vi "YokoGS200 CheckStatus.vi"(8 "error in (no error)":errorcluster, 11 "VISA Rsrc":refnum<visa-resource-name>="SR530") -> (0 "error out":errorcluster, 1 "Octet d'état":bool[](array[boolean]), 2 "octet d'état":u16, 3 "VISA Rsrc Out":refnum<visa-resource-name>="GPIB0::12::INSTR")   [LabVIEW 2012]
uses:
  <userlib>/Yoko GS200/YokoGS200 lvl_states ctl.ctl
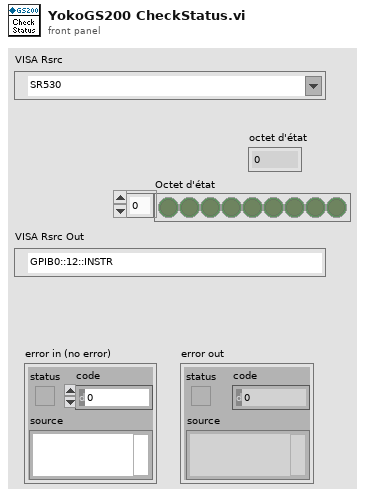
[diagram p1: front panel]
types:
  T1 = typedef "YokoGS200 lvl_states ctl.ctl" = enum16{"RampStep", "Send Command", "Check Errors", "End"}
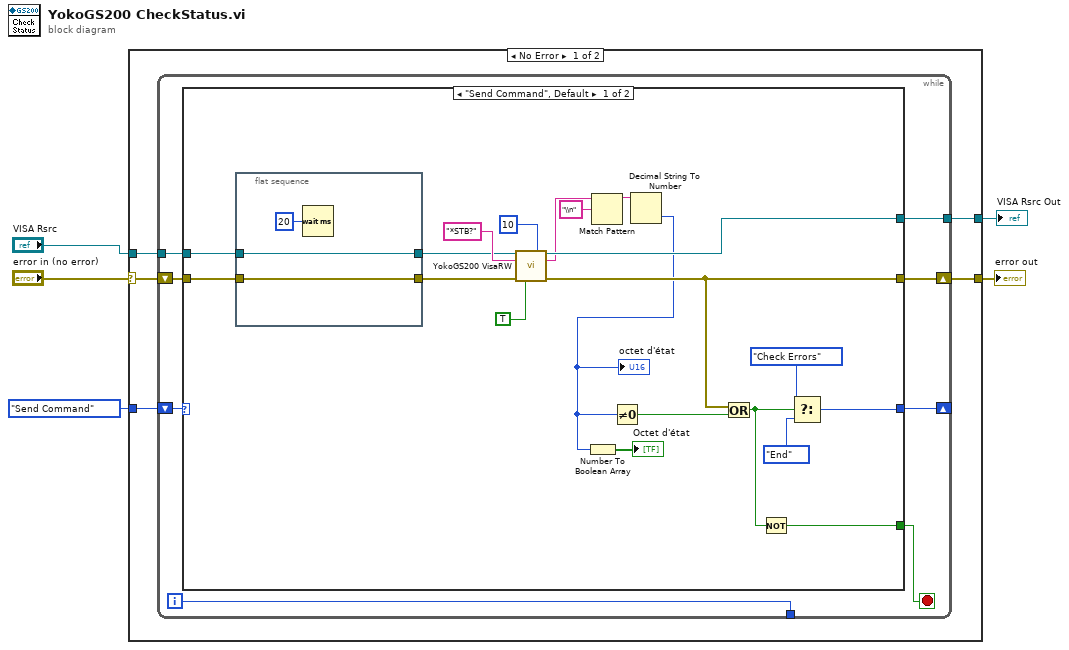
[diagram p0: block diagram]
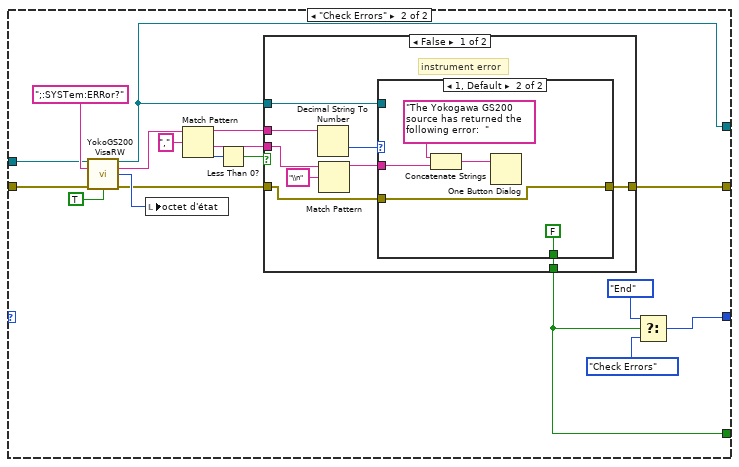
[diagram p2: hidden frame]
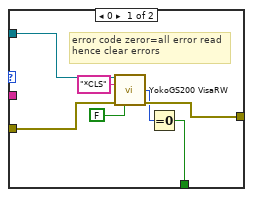
[diagram p3: hidden frame]
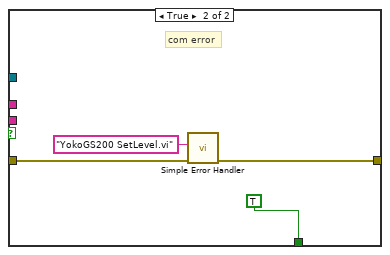
[diagram p4: hidden frame]
diagram:
  n1 = case shown="No Error" "error in (no error)" {
    selector: "error in (no error)" -> [w10 w85]
    tunnel: "VISA Rsrc" -> [w9 w86]
    tunnel: [w6 w85] -> w3
    tunnel: [w8 w86] -> w2
    tunnel: YokoGS200_lvl_states_ctl."Send Command" ("Level State") -> [w7 _]
    frame No Error {
      n2 = while {
        tunnel: w9 -> [w17]
        tunnel: [w16] -> w8
        shift-right: [w14] -> _
        shift-left: w7 -> [w15]
        shift-right: [w12] -> w6
        shift-left: w10 -> [w18]
        tunnel: [w11] -> _
        i -> [w11]
        stop <- w13 stop-if-true
        n3 = case shown="\"Send Command\", Default" w15 {
          tunnel: w18 -> [w21 w42]
          tunnel: w17 -> [w22 w48]
          tunnel: [w38 w45] -> w16
          tunnel: [w36 w44] -> w12
          tunnel: [w35 w50] -> w14
          tunnel: [w31 w43] -> w13
          frame "Send Command", Default {
            n4 = flat-sequence {
              tunnel: [w41] -> w20
              tunnel: w21 -> [w41]
              tunnel: [w40] -> w19
              tunnel: w22 -> [w40]
              frame #0 {
                n5 = Wait (ms)(milliseconds to wait=u32 20) -> ()  [unwired: 1 out]
              }
            }
            n6 = call <userlib>:"YokoGS200 VisaRW.vi"("VISA Rsrc"=w19, "Délais (0 ms)"=u32 10, "ChaineCom"="*STB?" ("string"), "error in (no error)"=w20, "Lecture?(T)"=TRUE) -> ("VISA Rsrc Out"=w38:refnum<visa-resource-name>, "ChaineRep"=w28:string, "error out"=w36:errorcluster)  [unwired: 6 in, 2 out]
            n7 = Match Pattern(string=w28, regular expression="\\n") -> (before substring=w26:string)  [unwired: 1 in, 3 out]
            n8 = Decimal String To Number(string=w26) -> (number=w25:i32)  [unwired: 2 in, 1 out]
            "octet d'état" <- w25
            n9 = Number To Boolean Array(number=w25) -> (Boolean array=→"Octet d'état":bool[])
            n10 = Not Equal To 0?(x=w25) -> (x != 0?=w37:bool)
            n11 = Or(x=w36, y=w37) -> (x .or. y?=w32:bool)
            n12 = Not(x=w32) -> (.not. x?=w31:bool)
            n13 = Select(t=YokoGS200_lvl_states_ctl."Check Errors" ("Level State"), s=w32, f=YokoGS200_lvl_states_ctl."End" ("Level State")) -> (s? t:f=w35:T1)
          }
          frame "Check Errors" {
            n14 = call <userlib>:"YokoGS200 VisaRW.vi"("VISA Rsrc"=w48, "ChaineCom"=";:SYSTem:ERRor?" ("initial string"), "error in (no error)"=w42, "Poll?(F)"=TRUE) -> ("VISA Rsrc Out"=w45:refnum<visa-resource-name>, "ChaineRep"=w55:string, "octet d'état"=w49:u16, "error out"=w46:errorcluster)  [unwired: 7 in, 1 out]
            n15 = local write "octet d'état"(w49) -> ()
            n16 = Match Pattern(string=w55, regular expression=",") -> (before substring=w58:string, after substring=w47:string, offset past match=w54:i32)  [unwired: 1 in, 1 out]
            n17 = Less Than 0?(x=w54) -> (x < 0?=w53:bool)
            n18 = case shown="False" w53 {
              tunnel: w58 -> [w68 _]
              tunnel: w47 -> [w67 _]
              tunnel: [w64 TRUE] -> w43
              tunnel: w46 -> [w63 w83]
              tunnel: w45 -> [w62 _]
              tunnel: [w61 w81] -> w44
              frame False {
                # "instrument error"
                n19 = Decimal String To Number(string=w68) -> (number=w60:i32)  [unwired: 2 in, 1 out]
                n20 = Match Pattern(string=w67, regular expression="\\n") -> (before substring=w65:string)  [unwired: 1 in, 3 out]
                n21 = case shown="1, Default" w60 {
                  tunnel: w65 -> [_ w78]
                  tunnel: [w69 FALSE] -> w64
                  tunnel: w63 -> [w75 w76]
                  tunnel: w62 -> [w74 _]
                  tunnel: [w73 w76] -> w61
                  frame 0 {
                    # "error code zeror=all error read\nhence clear errors"
                    n22 = call <userlib>:"YokoGS200 VisaRW.vi"("VISA Rsrc"=w74, "ChaineCom"="*CLS", "error in (no error)"=w75, "Lecture?(T)"=FALSE) -> ("octet d'état"=w70:u16, "error out"=w73:errorcluster)  [unwired: 7 in, 3 out]
                    n23 = Equal To 0?(x=w70) -> (x = 0?=w69:bool)
                  }
                  frame 1, Default {
                    n24 = Concatenate Strings("The Yokogawa GS200 source has returned the following error:  ", w78) -> (w80:string)
                    n25 = One Button Dialog(message=w80) -> ()  [unwired: 1 in, 1 out]
                  }
                }
              }
              frame True {
                # "com error"
                n26 = call <vilib>:"Simple Error Handler.vi"("error source (\" \")"="YokoGS200 SetLevel.vi" ("error source (\" \")"), "error in (no error)"=w83) -> ("error out"=w81:errorcluster)  [unwired: 3 in, 4 out]
              }
            }
            n27 = Select(t=YokoGS200_lvl_states_ctl."End" ("Level State"), s=w43, f=YokoGS200_lvl_states_ctl."Check Errors" ("Level State")) -> (s? t:f=w50:T1)
          }
        }
      }
    }
    frame Error {
    }
  }
  "error out" <- w3
  "VISA Rsrc Out" <- w2
